vi "Read avg_rating.vi"(8 "error in (no error)":errorcluster, 11 "Package in":refnum<class "Package.lvclass">) -> (0 "error out":errorcluster, 2 "avg_rating":i32, 3 "Package out":refnum<class "Package.lvclass">)   [LabVIEW 2017, in "GCentral API.lvlib" / "Package.lvclass"]
uses:
  Package.lvclass
  Package.lvclass/Package.ctl
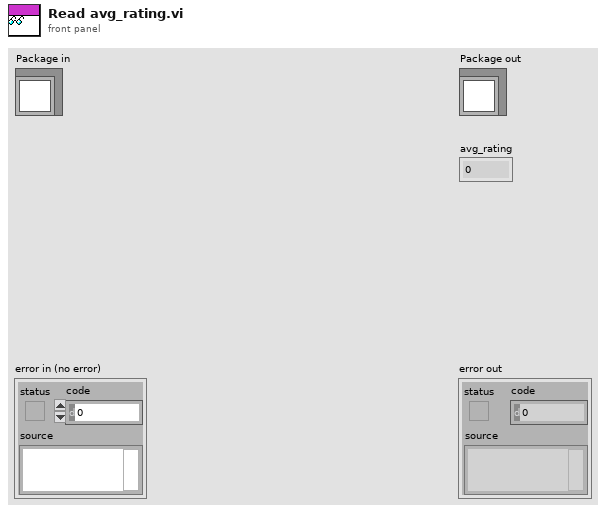
[diagram p1: front panel]
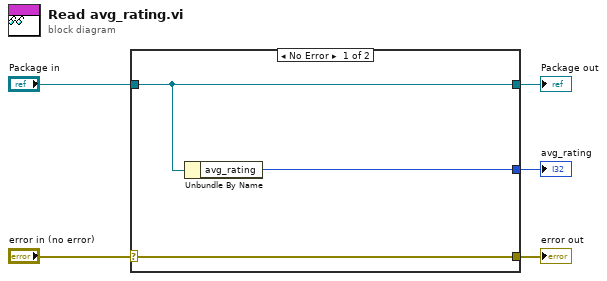
[diagram p0: block diagram]
diagram:
  n1 = case shown="No Error" "error in (no error)" {
    selector: "error in (no error)" -> [w8 w9]
    tunnel: [w8 w9] -> w4
    tunnel: [w7 w10] -> w2
    tunnel: "Package in" -> [w7 w10]
    tunnel: [w6 _] -> w1
    frame No Error {
      n2 = Unbundle By Name(w7) -> ("avg_rating"=w6:i32)
    }
    frame Error {
    }
  }
  "error out" <- w4
  "Package out" <- w2
  "avg_rating" <- w1
